vi "HDI-BBM Geometry Definition Acquire.vi"() -> ()   [LabVIEW 2011]
uses:
  Shared Components/Orient3d Class/Type Definitions/Quaternion.ctl
  Shared Components/Config Manager Class/Type Definitions/Part Type.ctl
  Shared Components/Config Manager Class/Type Definitions/Camera Enum.ctl
  Shared Components/Gantry Class/Gantry Class.lvclass
  Shared Components/CameraTool Class/CameraTool Class.lvclass
  Shared Components/Vec3d Class/Vec3d Class.lvclass
  Shared Components/Orient3d Class/Orient3d Class.lvclass
  Shared Components/Config Manager Class/Config Manager Class.lvclass
panel:
  in  "Part Type":T1
  out "Fit Residual":dbl
  out "Part Orientation":T2
  out "Part Center":cluster{"X":dbl, "Y":dbl, "Z":dbl}
  out "Stop":bool=TRUE
  out "Local Position":cluster{"X":dbl, "Y":dbl, "Z":dbl}
  out "preview":T3(plugin-control)
  out "Global Position":cluster{"X":dbl, "Y":dbl, "Z":dbl}
  in  "Slot":i32
  in  "Config Folder":path=path "C:/Users/Husker/Desktop/gantry/Config"
  in  "Chuck":i32=1
  # "INSTRUCTIONS\n==========\nThis is a tool to help in the acquisition\nof geometry definitions i.e. the local positions\nof feature points on parts.\n\nBegin by setting appropriate values in the \nlower left corner.\n\nThen use the MPG(hand control) to move\nto the feature positions of interest. The gantry's\n\"global\" position and the corresponding part's\n\"local\" position can be read off from the below\nindicators.\n\nSimply click the x in the top right corner to quit"
  # "Set this to the appropriate slot number(0-3) before running"
  # "Set this to the appropriate chuck number(0-4) before running"
  # "Set this to the appropriate part type (HDI, BBM, etc.) before running"
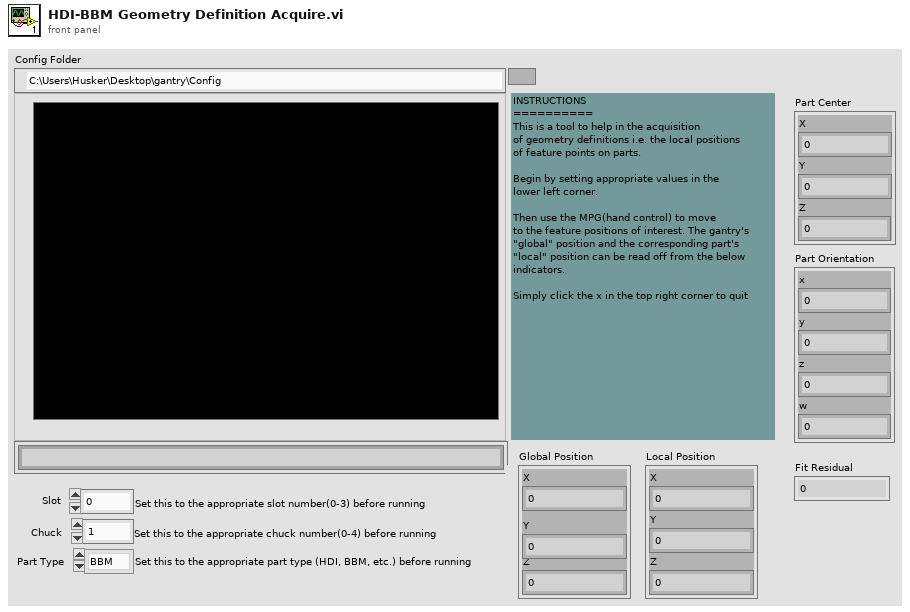
[diagram p1: front panel]
types:
  T1 = typedef "Part Type.ctl" = enum16{"BBM", "HDI", "GLUERESERVOIR", "STAMP", "WEIGHT"}
  T2 = typedef "Quaternion.ctl" = cluster{"x":dbl, "y":dbl, "z":dbl, "w":dbl}
  T3 = typedef "IMAQ Image.ctl" = refnum<image>
  T4 = typedef "Image Type" = u32
  T5 = typedef "Fiducial Image.ctl" = cluster{"Fiducial Image":T6, "Selected Fiducial":T7, "fiducial name":string}
  T6 = typedef "Physical Image.ctl" = cluster{"Image Position":refnum<class "Vec3d Class.lvclass">, "Image Reference":T3, "Field of View":cluster{"x(mm)":dbl, "y(mm)":dbl}}
  T7 = typedef "Fiducial with Source.ctl" = cluster{"Fiducial Image Coordinate":refnum<class "Vec3d Class.lvclass">, "Fiducial Source":enum16{"Pattern Recognition", "User", "Error", "Default"}}
  T8 = cluster{"fiducial location":refnum<class "Vec3d Class.lvclass">, "fiducial name":string}
  T9 = typedef "Fiducial Type.ctl" = enum16{"HDI", "BBM"}
  T10 = cluster{"Feature Coordinates":refnum<class "Vec3d Class.lvclass">, "Feature Name":string}[]
  T11 = typedef "Position_Orientation.ctl" = cluster{"Center":refnum<class "Vec3d Class.lvclass">, "Orientation":refnum<class "Orient3d Class.lvclass">}
  T12 = typedef "Camera Enum.ctl" = enum16{"GANTRY HEAD", "NEEDLE CALIBRATION X", "NEEDLE CALIBRATION Y"}
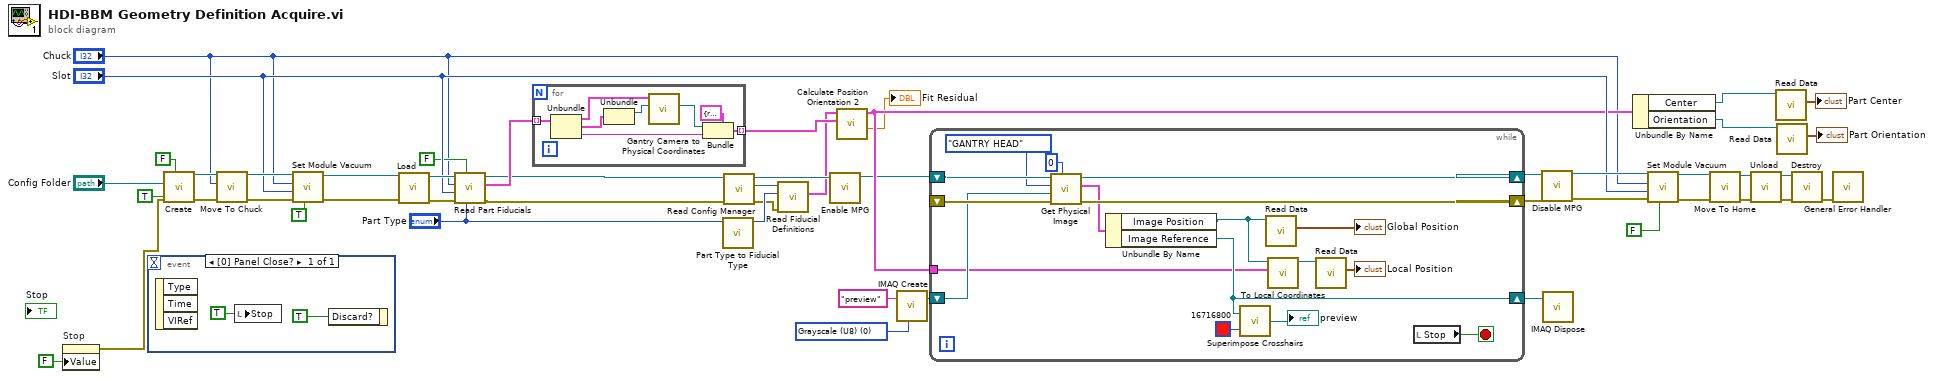
[diagram p0: block diagram]
diagram:
  w37 = T4 0 items=["Grayscale (U8)", "Grayscale (I16)", "Grayscale (SGL)", "Complex (CSG)", "RGB (U32)", "HSL (U32)", "RGB (U64)", "Grayscale (U16)"] ("Image Type")
  n1 = property on="Stop" class="Bool (strict)"("Value"=FALSE ("Stop")) -> (error out=w29:errorcluster)  [unwired: 2 in, 1 out]
  n2 = event shown="[0] Panel Close?" {
    selector: _ -> [_]
    dyn-events: _ -> [_]
    timeout: _ -> [_]
    event Panel Close? {
      n3 = event-data() -> ()  [unwired: 1 in, 3 out]
      n4 = local write "Stop"(TRUE ("Stop")) -> ()
      n5 = event-data("Discard?"=TRUE) -> ()  [unwired: 1 in, 1 out]
    }
  }
  n6 = call "Create.vi"("Virtual Mode"=FALSE, "error in"=w29, "HOME?"=TRUE, "Config Folder"="Config Folder") -> ("error out"=w48:errorcluster, "Gantry out"=w46:refnum<class "Gantry Class.lvclass">)  [unwired: 6 in]
  n7 = call-dynamic "Move To Chuck.vi"("error in"=w48, "Chuck"="Chuck", "Gantry in"=w46) -> ("error out"=w47:errorcluster, "Gantry out"=w45:refnum<class "Gantry Class.lvclass">)  [unwired: 7 in]
  n8 = call-dynamic "Set Module Vacuum.vi"("On/Off"=TRUE, "error in"=w47, "Slot Number"="Slot", "Chuck Number"="Chuck", "Gantry in"=w45) -> ("error out"=w16:errorcluster, "Gantry out"=w17:refnum<class "Gantry Class.lvclass">)  [unwired: 5 in]
  n9 = call "Load.vi"("error in"=w16, "Gantry In"=w17) -> ("error out"=w26:errorcluster, "CameraTool out"=w27:refnum<class "CameraTool Class.lvclass">)  [unwired: 8 in]
  n10 = call-dynamic "Read Part Fiducials.vi"("Part Type"="Part Type", "Dispose Images?"=FALSE, "error in"=w26, "Slot"="Slot", "Chuck"="Chuck", "CameraTool in"=w27) -> ("error out"=w12:errorcluster, "Fiducials"=w23:T5[], "CameraTool out"=w13:refnum<class "CameraTool Class.lvclass">)  [unwired: 3 in]
  n11 = for {
    tunnel: w23 -> [w60] mode=indexing
    tunnel: [w53] -> w22 mode=indexing
    n12 = Unbundle(w60) -> ("Fiducial Image"=w57:T6, "Selected Fiducial"=w56:T7, "fiducial name"=w58:string)
    n13 = Unbundle(w56) -> ("Fiducial Image Coordinate"=w55:refnum<class "Vec3d Class.lvclass">)  [unwired: 1 out]
    n14 = call "Gantry Camera to Physical Coordinates.vi"("Image Coordinate"=w55, "Physical Image"=w57) -> ("Global Coordinate"=w54:refnum<class "Vec3d Class.lvclass">)  [unwired: 7 in, 2 out]
    n15 = Bundle(cluster=T8 {"fiducial location"=refnum, "fiducial name"=""} ("fiducial with name"), "fiducial location"=w54, "fiducial name"=w58) -> (w53:T8)
  }
  n16 = call "Part Type to Fiducial Type.vi"("Part Type"="Part Type") -> ("Fiducial Type"=w8:T9)  [unwired: 9 in, 1 out]
  n17 = call-dynamic "Read Config Manager.vi"("error in"=w12, "Gantry in"=w13) -> ("error out"=w7:errorcluster, "Config Manager"=w10:refnum<class "Config Manager Class.lvclass">, "Gantry out"=w11:refnum<class "CameraTool Class.lvclass">)  [unwired: 7 in]
  n18 = call "Read Fiducial Definitions.vi"("error in"=w7, "Fiducial Type"=w8, "Config Manager in"=w10) -> ("Feature Definitions"=w6:T10)  [unwired: 6 in, 2 out]
  n19 = call-dynamic "Enable MPG.vi"("Gantry in"=w11) -> ("Gantry out"=w15:refnum<class "CameraTool Class.lvclass">)  [unwired: 9 in, 1 out]
  n20 = call "Calculate Position Orientation 2.vi"("Measured Global Positions"=w22, "Known Local Positions"=w6) -> ("Residual"=→"Fit Residual":dbl, "PositionOrientation"=w20:T11)  [unwired: 7 in, 1 out]
  n21 = call "IMAQ Create"("Image Name"="preview", "Image Type"=w37) -> ("New Image"=w36:T3)  [unwired: 3 in, 1 out]
  n22 = while {
    shift-right: [w70] -> w33
    shift-left: _ -> [w76]
    shift-right: [w71] -> w34
    shift-left: w15 -> [w77]
    shift-right: [w68] -> w35
    shift-left: w36 -> [w72]
    tunnel: w20 -> [w63]
    stop <- w64 stop-if-true
    n23 = call-dynamic "Get Physical Image.vi"("Delay(milliseconds)"=0, "error in"=w76, "Image In"=w72, "Camera Name"=Camera_Enum."GANTRY HEAD", "Gantry in"=w77) -> ("error out"=w70:errorcluster, "Physical Image"=w69:T6, "Gantry out"=w71:refnum<class "CameraTool Class.lvclass">)  [unwired: 4 in]
    n24 = Unbundle By Name(w69) -> ("Image Position"=w67:refnum<class "Vec3d Class.lvclass">, "Image Reference"=w68:T3)
    n25 = call "Superimpose Crosshairs.vi"("Grid Line Color"=u32 16716800, "Refnum in"=w68) -> ("Refnum out"=→"preview":T3)
    n26 = call-dynamic "Read Data.vi"("Vec3d Class in"=w67) -> ("Data"=→"Global Position":cluster{"X":dbl, "Y":dbl, "Z":dbl})  [unwired: 8 in, 2 out]
    n27 = call "To Local Coordinates.vi"("Center/Orientation"=w63, "Global Coordinates"=w67) -> ("Local Coordinates"=w66:refnum<class "Vec3d Class.lvclass">)  [unwired: 8 in, 1 out]
    n28 = call-dynamic "Read Data.vi"("Vec3d Class in"=w66) -> ("Data"=→"Local Position":cluster{"X":dbl, "Y":dbl, "Z":dbl})  [unwired: 8 in, 2 out]
    n29 = local read "Stop"() -> (w64:bool)
  }
  n30 = call-dynamic "Disable MPG.vi"("error in"=w33, "Gantry in"=w34) -> ("error out"=w42:errorcluster, "Gantry out"=w43:refnum<class "CameraTool Class.lvclass">)  [unwired: 8 in]
  n31 = call "IMAQ Dispose"("Image"=w35) -> ()  [unwired: 5 in, 1 out]
  n32 = Unbundle By Name(w20) -> ("Center"=w19:refnum<class "Vec3d Class.lvclass">, "Orientation"=w18:refnum<class "Orient3d Class.lvclass">)
  n33 = call-dynamic "Set Module Vacuum.vi"("On/Off"=FALSE, "error in"=w42, "Slot Number"="Slot", "Chuck Number"="Chuck", "Gantry in"=w43) -> ("error out"=w40:errorcluster, "Gantry out"=w41:refnum<class "CameraTool Class.lvclass">)  [unwired: 5 in]
  n34 = call-dynamic "Move To Home.vi"("error in"=w40, "Gantry in"=w41) -> ("error out"=w3:errorcluster, "Gantry out"=w4:refnum<class "CameraTool Class.lvclass">)  [unwired: 8 in]
  n35 = call "Unload.vi"("error in"=w3, "CameraTool in"=w4) -> ("error out"=w1:errorcluster, "Gantry out"=w2:refnum<class "Gantry Class.lvclass">)  [unwired: 8 in]
  n36 = call-dynamic "Read Data.vi"("Vec3d Class in"=w19) -> ("Data"=→"Part Center":cluster{"X":dbl, "Y":dbl, "Z":dbl})  [unwired: 8 in, 2 out]
  n37 = call "Read Data.vi"("Orient3d in"=w18) -> ("Quaternion"=→"Part Orientation":T2)  [unwired: 8 in, 2 out]
  n38 = call "Destroy.vi"("error in"=w1, "Gantry Class in"=w2) -> ("error out"=w32:errorcluster)  [unwired: 9 in]
  n39 = call <vilib>:"General Error Handler.vi"("error in (no error)"=w32) -> ()  [unwired: 10 in, 5 out]
